vi "newDevice.vi"(8 "error in (no error)":errorcluster, 9 "details":T2, 10 "Device Type":T1=enum."k4b2", 11 "reference in":refnum<class "Devices Controller.lvclass">) -> (0 "error out":errorcluster, 3 "reference out":refnum<class "Devices Controller.lvclass">)   [LabVIEW 2015, in "Devices Controller.lvclass"]
uses:
  Devices Controller.lvclass
  deviceType.ctl
  APP/excelFile_class/fileType.ctl
  APP/k4b2_class/k4b2.lvclass
  APP/rmr_class/rmr.lvclass
  APP/fitmate_class/fitmate.lvclass
  APP/cpet_class/cpet.lvclass
  APP/bodpod_class/bodpod.lvclass
  APP/peapod_class/peapod.lvclass
  APP/excelFile_class/excelFile.lvclass
  File Controller_llb/File Controller.lvclass
  APP/k5_class/k5.lvclass
  APP/bb-pft_class/bb-pft.lvclass
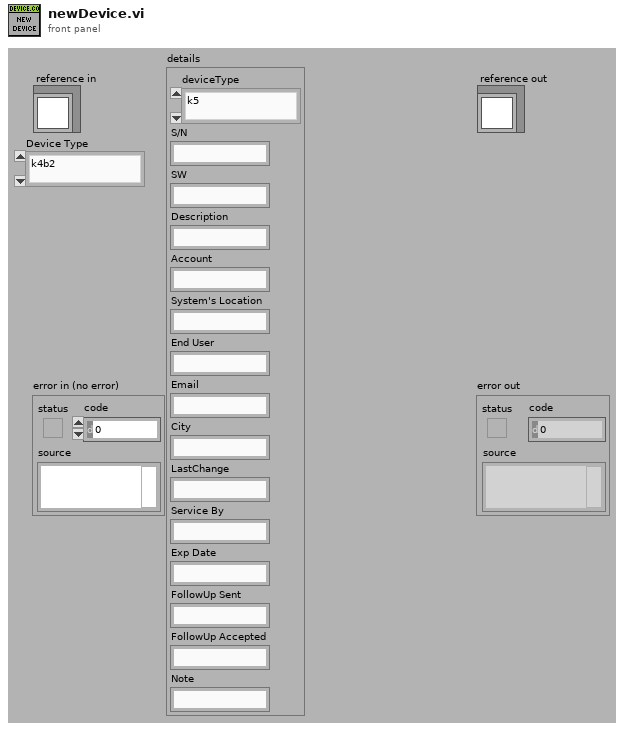
[diagram p1: front panel]
types:
  T1 = typedef "Devices Controller.lvclass/deviceType.ctl" = enum16{"k5", "k4b2", "fitmate", "cpet", "rmr", "bodyBoxPft", "bp", "pp"}
  T2 = cluster{"deviceType":T1, "S/N":string, "SW":string, "Description":string, "Account":string, "System's Location":string, "End User":string, "Email":string, "City":string, "LastChange":string, "Service By":string, "Exp Date":string, "FollowUp Sent":string, "FollowUp Accepted":string, "Note":string}
  T3 = typedef "excelFile.lvclass/fileType.ctl" = enum16{"devices", "items", "partsTracking"}
  T4 = cluster{"deviceType":T1, "S/N":string, "SW":string, "Description":string, "Account":string, "System's Location":string, "End User":string, "Email":string, "City":string, "FollowUp Sent":string, "FollowUp Accepted":string, "Note":string}
  T5 = typedef "Devices Controller.lvclass/ObjectAttributesRef.ctl" = refnum<data-value>
  T6 = typedef "Devices Controller.lvclass/ObjectAttributes.ctl" = cluster{"MyAttribute":dbl, "file_controller_ref":refnum<class "File Controller.lvclass">, "data":string[][][], "devices_refs":cluster{"k4b2_refs":refnum<class "k4b2.lvclass">[], "rmr_refs":refnum<class "rmr.lvclass">[], "bod_pod_refs":refnum<class "bodpod.lvclass">[], "cpet_refs":refnum<class "cpet.lvclass">[], "fitmate_refs":refnum<class "fitmate.lvclass">[], "pea_pod_refs":refnum<class "peapod.lvclass">[], "k5_refs":refnum<class "k5.lvclass">[], "bb-pft_refs":refnum<class "bb-pft.lvclass">[]}}
  T7 = cluster{"k4b2_refs":refnum<class "k4b2.lvclass">[], "rmr_refs":refnum<class "rmr.lvclass">[], "bod_pod_refs":refnum<class "bodpod.lvclass">[], "cpet_refs":refnum<class "cpet.lvclass">[], "fitmate_refs":refnum<class "fitmate.lvclass">[], "pea_pod_refs":refnum<class "peapod.lvclass">[], "k5_refs":refnum<class "k5.lvclass">[], "bb-pft_refs":refnum<class "bb-pft.lvclass">[]}
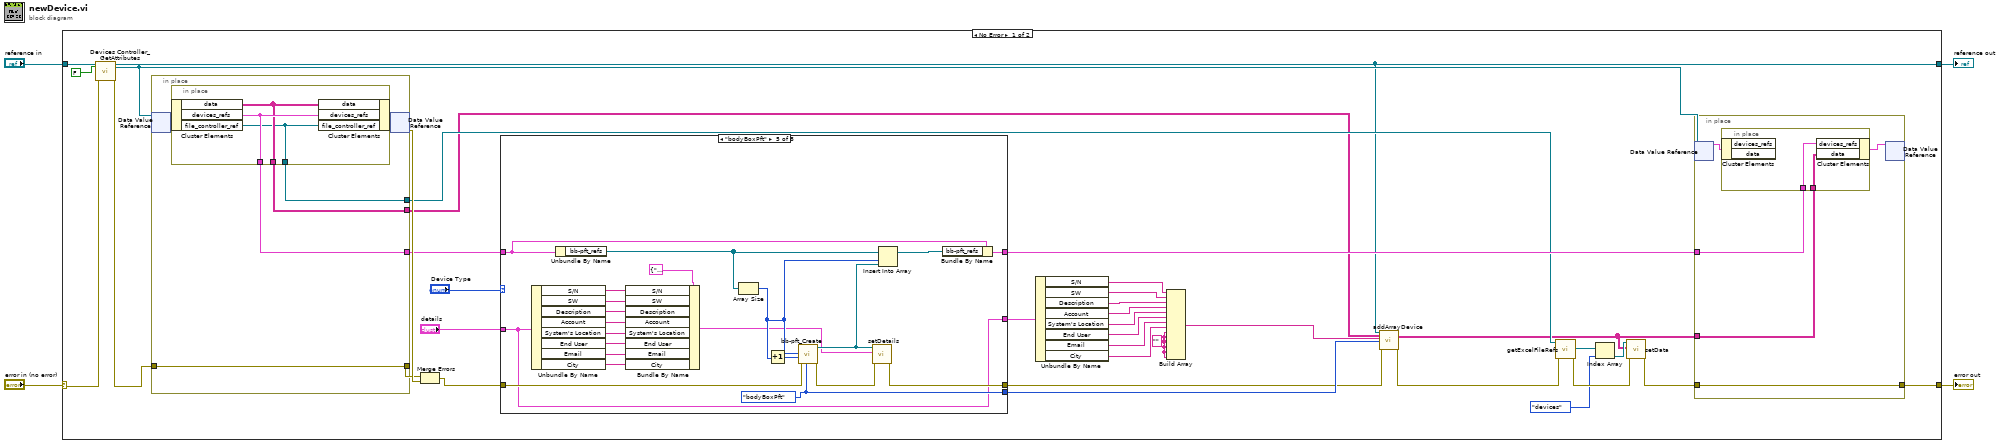
[diagram p0: block diagram]
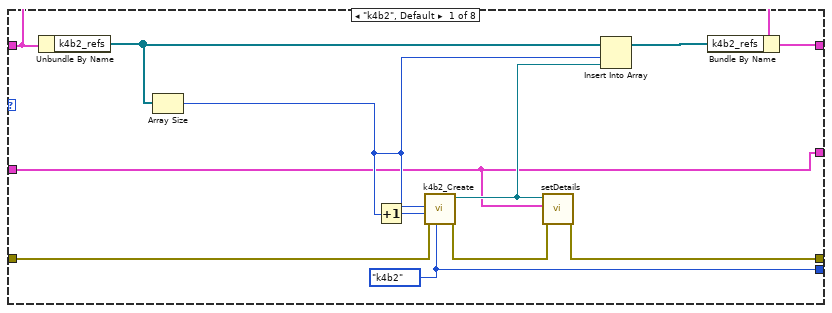
[diagram p2: hidden frame]
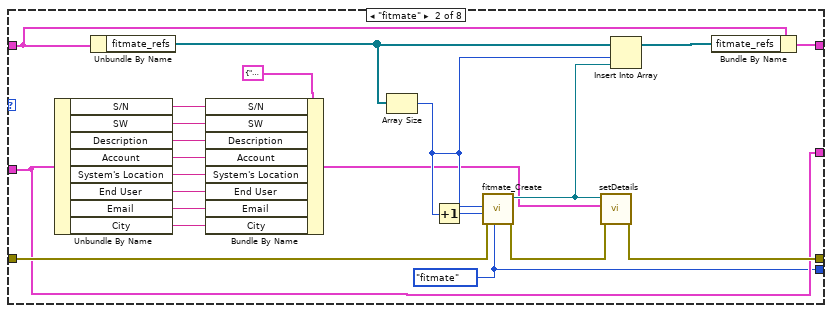
[diagram p3: hidden frame]
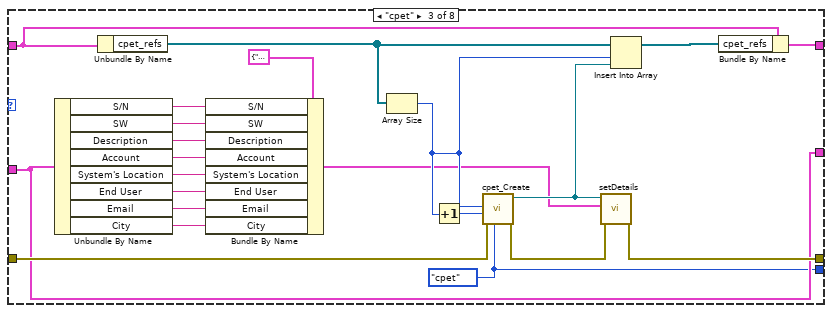
[diagram p4: hidden frame]
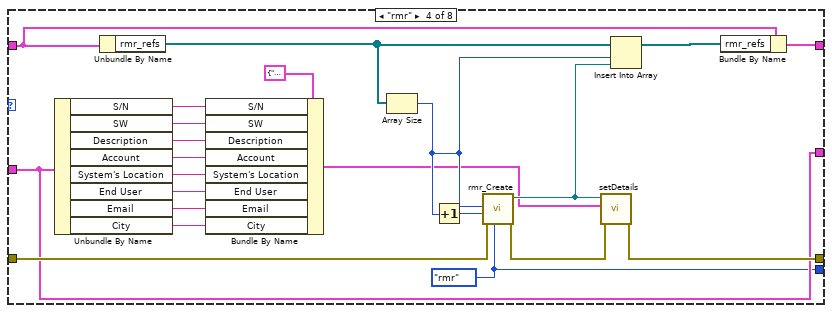
[diagram p5: hidden frame]
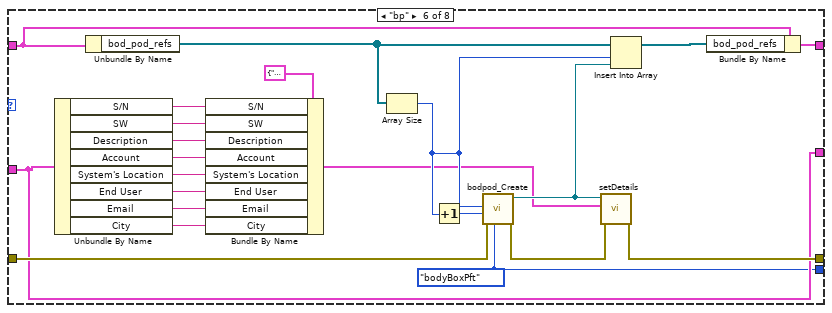
[diagram p6: hidden frame]
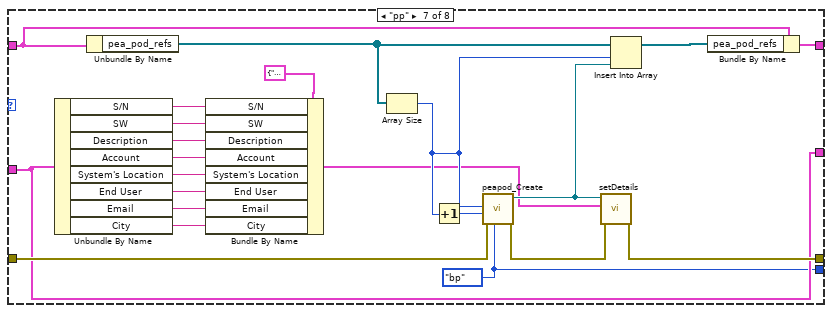
[diagram p7: hidden frame]
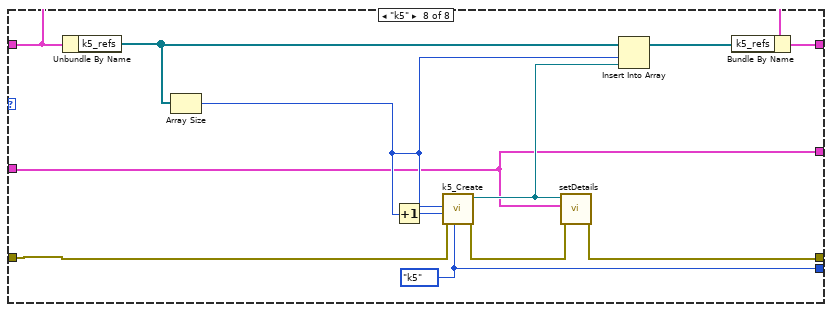
[diagram p8: hidden frame]
diagram:
  n1 = case shown="No Error" "error in (no error)" {
    selector: "error in (no error)" -> [w36 w214]
    tunnel: [w31 w214] -> w3
    tunnel: [w5 w213] -> w1
    tunnel: "reference in" -> [w38 w213]
    frame No Error {
      w10 = "" ("City")
      n2 = call "Devices Controller_GetAttributes.vi"("reference in"=w38, "return data? (T)"=FALSE, "error in (no error)"=w36) -> ("reference out"=w5:refnum<class "Devices Controller.lvclass">, "attributes ref"=w30:T5, "error out"=w32:errorcluster)  [unwired: 13 in, 1 out]
      n3 = in-place {
        in-place-border: w32 -> [w207]
        in-place-border: [w207] -> w39
        in-place-border: [w206] -> w33
        in-place-border: [w205] -> w9
        in-place-border: [w204] -> w14
        n4 = in-place-dvr #1(w30) -> (w208:T6)  [unwired: 1 out]
        n5 = in-place {
          in-place-border: [w212] -> w206
          in-place-border: [w211] -> w205
          in-place-border: [w210] -> w204
          n6 = in-place-cluster #2(w208) -> ("data"=w211:string[][][], "devices_refs"=w212:T7, "file_controller_ref"=w210:refnum<class "File Controller.lvclass">)
          n7 = in-place-cluster #2("data"=w211, "devices_refs"=w212, "file_controller_ref"=w210) -> (w209:T6)
        }
        n8 = in-place-dvr #1(w209) -> (w40:errorcluster)  [unwired: 1 out]
      }
      n9 = Merge Errors(w39, w40) -> (w35:errorcluster)
      n10 = case shown="\"bodyBoxPft\"" "Device Type" {
        tunnel: w35 -> [w59 w75 w97 w119 w132 w163 w185 w197]
        tunnel: [w50 w74 w96 w118 w130 w162 w184 w196] -> w7
        tunnel: "details" -> [w48 w63 w85 w107 w126 w151 w173 w195]
        tunnel: w33 -> [w56 w72 w94 w116 w131 w160 w182 w198]
        tunnel: [w51 w73 w95 w117 w129 w161 w183 w194] -> w29
        tunnel: [w48 w63 w85 w107 w126 w151 w173 w195] -> w17
        tunnel: [w49 w62 w84 w106 w127 w150 w172 w193] -> w11
        frame "k4b2", Default {
          w49 = deviceType."k4b2" ("deviceType")
          n11 = Unbundle By Name(w56) -> ("k4b2_refs"=w55:refnum<class "k4b2.lvclass">[])
          n12 = Array Size(array=w55) -> (size(s)=w52:i32)
          n13 = Increment(x=w52) -> (x+1=w58:i32)
          n14 = call "k4b2_Create.vi"("deviceType"=w49, "error in (no error)"=w59, "dim"=w58, "index"=w52) -> ("error out"=w57:errorcluster, "reference out"=w53:refnum<class "k4b2.lvclass">)  [unwired: 6 in]
          n15 = call "setDetails.vi"("error in (no error)"=w57, "details"=w48, "reference in"=w53) -> ("error out"=w50:errorcluster)  [unwired: 7 in, 1 out]
          n16 = Insert Into Array(array=w55, index=w52, new element=w53) -> (w54:refnum<class "k4b2.lvclass">[])
          n17 = Bundle By Name(cluster=w56, "k4b2_refs"=w54) -> (w51:T7)
        }
        frame "fitmate" {
          w62 = deviceType."fitmate" ("deviceType")
          n18 = Unbundle By Name(w63) -> ("S/N"=w71:string, "SW"=w70:string, "Description"=w69:string, "Account"=w68:string, "System's Location"=w67:string, "End User"=w66:string, "Email"=w65:string, "City"=w64:string)
          n19 = Unbundle By Name(w72) -> ("fitmate_refs"=w79:refnum<class "fitmate.lvclass">[])
          n20 = Bundle By Name(cluster=T4 {"deviceType"=enum."k5", "S/N"="", "SW"="", "Description"="", "Account"="", "System's Location"="", "End User"="", "Email"="", "City"="", "FollowUp Sent"="", "FollowUp Accepted"="", "Note"=""} ("details"), "S/N"=w71, "SW"=w70, "Description"=w69, "Account"=w68, "System's Location"=w67, "End User"=w66, "Email"=w65, "City"=w64) -> (w60:T4)
          n21 = Array Size(array=w79) -> (size(s)=w76:i32)
          n22 = Increment(x=w76) -> (x+1=w81:i32)
          n23 = call "fitmate_Create.vi"("deviceType"=w62, "error in (no error)"=w75, "dim"=w81, "index"=w76) -> ("error out"=w80:errorcluster, "reference out"=w77:refnum<class "fitmate.lvclass">)  [unwired: 6 in]
          n24 = call "setDetails.vi"("error in (no error)"=w80, "details"=w60, "reference in"=w77) -> ("error out"=w74:errorcluster)  [unwired: 7 in, 1 out]
          n25 = Insert Into Array(array=w79, index=w76, new element=w77) -> (w78:refnum<class "fitmate.lvclass">[])
          n26 = Bundle By Name(cluster=w72, "fitmate_refs"=w78) -> (w73:T7)
        }
        frame "cpet" {
          w84 = deviceType."cpet" ("deviceType")
          n27 = Unbundle By Name(w85) -> ("S/N"=w93:string, "SW"=w92:string, "Description"=w91:string, "Account"=w90:string, "System's Location"=w89:string, "End User"=w88:string, "Email"=w87:string, "City"=w86:string)
          n28 = Unbundle By Name(w94) -> ("cpet_refs"=w101:refnum<class "cpet.lvclass">[])
          n29 = Bundle By Name(cluster=T4 {"deviceType"=enum."k5", "S/N"="", "SW"="", "Description"="", "Account"="", "System's Location"="", "End User"="", "Email"="", "City"="", "FollowUp Sent"="", "FollowUp Accepted"="", "Note"=""} ("details"), "S/N"=w93, "SW"=w92, "Description"=w91, "Account"=w90, "System's Location"=w89, "End User"=w88, "Email"=w87, "City"=w86) -> (w82:T4)
          n30 = Array Size(array=w101) -> (size(s)=w98:i32)
          n31 = Increment(x=w98) -> (x+1=w103:i32)
          n32 = call "cpet_Create.vi"("deviceType"=w84, "error in (no error)"=w97, "dim"=w103, "index"=w98) -> ("error out"=w102:errorcluster, "reference out"=w99:refnum<class "cpet.lvclass">)  [unwired: 6 in]
          n33 = call "setDetails.vi"("error in (no error)"=w102, "details"=w82, "reference in"=w99) -> ("error out"=w96:errorcluster)  [unwired: 7 in, 1 out]
          n34 = Insert Into Array(array=w101, index=w98, new element=w99) -> (w100:refnum<class "cpet.lvclass">[])
          n35 = Bundle By Name(cluster=w94, "cpet_refs"=w100) -> (w95:T7)
        }
        frame "rmr" {
          w106 = deviceType."rmr" ("deviceType")
          n36 = Unbundle By Name(w107) -> ("S/N"=w115:string, "SW"=w114:string, "Description"=w113:string, "Account"=w112:string, "System's Location"=w111:string, "End User"=w110:string, "Email"=w109:string, "City"=w108:string)
          n37 = Unbundle By Name(w116) -> ("rmr_refs"=w123:refnum<class "rmr.lvclass">[])
          n38 = Bundle By Name(cluster=T4 {"deviceType"=enum."k5", "S/N"="", "SW"="", "Description"="", "Account"="", "System's Location"="", "End User"="", "Email"="", "City"="", "FollowUp Sent"="", "FollowUp Accepted"="", "Note"=""} ("details"), "S/N"=w115, "SW"=w114, "Description"=w113, "Account"=w112, "System's Location"=w111, "End User"=w110, "Email"=w109, "City"=w108) -> (w104:T4)
          n39 = Array Size(array=w123) -> (size(s)=w120:i32)
          n40 = Increment(x=w120) -> (x+1=w125:i32)
          n41 = call "rmr_Create.vi"("deviceType"=w106, "error in (no error)"=w119, "dim"=w125, "index"=w120) -> ("error out"=w124:errorcluster, "reference out"=w121:refnum<class "rmr.lvclass">)  [unwired: 6 in]
          n42 = call "setDetails.vi"("error in (no error)"=w124, "details"=w104, "reference in"=w121) -> ("error out"=w118:errorcluster)  [unwired: 7 in, 1 out]
          n43 = Insert Into Array(array=w123, index=w120, new element=w121) -> (w122:refnum<class "rmr.lvclass">[])
          n44 = Bundle By Name(cluster=w116, "rmr_refs"=w122) -> (w117:T7)
        }
        frame "bodyBoxPft" {
          w127 = deviceType."bodyBoxPft" ("deviceType")
          n45 = Unbundle By Name(w126) -> ("S/N"=w141:string, "SW"=w140:string, "Description"=w139:string, "Account"=w138:string, "System's Location"=w137:string, "End User"=w136:string, "Email"=w135:string, "City"=w134:string)
          n46 = Unbundle By Name(w131) -> ("bb-pft_refs"=w145:refnum<class "bb-pft.lvclass">[])
          n47 = Bundle By Name(cluster=T4 {"deviceType"=enum."k5", "S/N"="", "SW"="", "Description"="", "Account"="", "System's Location"="", "End User"="", "Email"="", "City"="", "FollowUp Sent"="", "FollowUp Accepted"="", "Note"=""} ("details"), "S/N"=w141, "SW"=w140, "Description"=w139, "Account"=w138, "System's Location"=w137, "End User"=w136, "Email"=w135, "City"=w134) -> (w128:T4)
          n48 = Array Size(array=w145) -> (size(s)=w142:i32)
          n49 = Increment(x=w142) -> (x+1=w147:i32)
          n50 = call "bb-pft_Create.vi"("deviceType"=w127, "error in (no error)"=w132, "dim"=w147, "index"=w142) -> ("error out"=w146:errorcluster, "reference out"=w143:refnum<class "bb-pft.lvclass">)  [unwired: 6 in]
          n51 = call "setDetails.vi"("error in (no error)"=w146, "details"=w128, "reference in"=w143) -> ("error out"=w130:errorcluster)  [unwired: 7 in, 1 out]
          n52 = Insert Into Array(array=w145, index=w142, new element=w143) -> (w144:refnum<class "bb-pft.lvclass">[])
          n53 = Bundle By Name(cluster=w131, "bb-pft_refs"=w144) -> (w129:T7)
        }
        frame "bp" {
          w150 = deviceType."bodyBoxPft" ("deviceType")
          n54 = Unbundle By Name(w151) -> ("S/N"=w159:string, "SW"=w158:string, "Description"=w157:string, "Account"=w156:string, "System's Location"=w155:string, "End User"=w154:string, "Email"=w153:string, "City"=w152:string)
          n55 = Unbundle By Name(w160) -> ("bod_pod_refs"=w167:refnum<class "bodpod.lvclass">[])
          n56 = Bundle By Name(cluster=T4 {"deviceType"=enum."k5", "S/N"="", "SW"="", "Description"="", "Account"="", "System's Location"="", "End User"="", "Email"="", "City"="", "FollowUp Sent"="", "FollowUp Accepted"="", "Note"=""} ("details"), "S/N"=w159, "SW"=w158, "Description"=w157, "Account"=w156, "System's Location"=w155, "End User"=w154, "Email"=w153, "City"=w152) -> (w148:T4)
          n57 = Array Size(array=w167) -> (size(s)=w164:i32)
          n58 = Increment(x=w164) -> (x+1=w169:i32)
          n59 = call "bodpod_Create.vi"("deviceType"=w150, "error in (no error)"=w163, "dim"=w169, "index"=w164) -> ("error out"=w168:errorcluster, "reference out"=w165:refnum<class "bodpod.lvclass">)  [unwired: 6 in]
          n60 = call "setDetails.vi"("error in (no error)"=w168, "details"=w148, "reference in"=w165) -> ("error out"=w162:errorcluster)  [unwired: 7 in, 1 out]
          n61 = Insert Into Array(array=w167, index=w164, new element=w165) -> (w166:refnum<class "bodpod.lvclass">[])
          n62 = Bundle By Name(cluster=w160, "bod_pod_refs"=w166) -> (w161:T7)
        }
        frame "pp" {
          w172 = deviceType."bp" ("deviceType")
          n63 = Unbundle By Name(w173) -> ("S/N"=w181:string, "SW"=w180:string, "Description"=w179:string, "Account"=w178:string, "System's Location"=w177:string, "End User"=w176:string, "Email"=w175:string, "City"=w174:string)
          n64 = Unbundle By Name(w182) -> ("pea_pod_refs"=w189:refnum<class "peapod.lvclass">[])
          n65 = Bundle By Name(cluster=T4 {"deviceType"=enum."k5", "S/N"="", "SW"="", "Description"="", "Account"="", "System's Location"="", "End User"="", "Email"="", "City"="", "FollowUp Sent"="", "FollowUp Accepted"="", "Note"=""} ("details"), "S/N"=w181, "SW"=w180, "Description"=w179, "Account"=w178, "System's Location"=w177, "End User"=w176, "Email"=w175, "City"=w174) -> (w170:T4)
          n66 = Array Size(array=w189) -> (size(s)=w186:i32)
          n67 = Increment(x=w186) -> (x+1=w191:i32)
          n68 = call "peapod_Create.vi"("deviceType"=w172, "error in (no error)"=w185, "dim"=w191, "index"=w186) -> ("error out"=w190:errorcluster, "reference out"=w187:refnum<class "peapod.lvclass">)  [unwired: 6 in]
          n69 = call "setDetails.vi"("error in (no error)"=w190, "details"=w170, "reference in"=w187) -> ("error out"=w184:errorcluster)  [unwired: 7 in, 1 out]
          n70 = Insert Into Array(array=w189, index=w186, new element=w187) -> (w188:refnum<class "peapod.lvclass">[])
          n71 = Bundle By Name(cluster=w182, "pea_pod_refs"=w188) -> (w183:T7)
        }
        frame "k5" {
          w193 = deviceType."k5" ("deviceType")
          n72 = Unbundle By Name(w198) -> ("k5_refs"=w201:refnum<class "k5.lvclass">[])
          n73 = Array Size(array=w201) -> (size(s)=w199:i32)
          n74 = Increment(x=w199) -> (x+1=w203:i32)
          n75 = call "k5_Create.vi"("deviceType"=w193, "error in (no error)"=w197, "dim"=w203, "index"=w199) -> ("error out"=w202:errorcluster, "reference out"=w200:refnum<class "k5.lvclass">)  [unwired: 6 in]
          n76 = call "setDetails.vi"("error in (no error)"=w202, "details"=w195, "reference in"=w200) -> ("error out"=w196:errorcluster)  [unwired: 7 in, 1 out]
          n77 = Insert Into Array(array=w201, index=w199, new element=w200) -> (w192:refnum<class "k5.lvclass">[])
          n78 = Bundle By Name(cluster=w198, "k5_refs"=w192) -> (w194:T7)
        }
      }
      n79 = Unbundle By Name(w17) -> ("S/N"=w28:string, "SW"=w27:string, "Description"=w26:string, "Account"=w25:string, "System's Location"=w24:string, "End User"=w23:string, "Email"=w22:string, "City"=w21:string)
      n80 = Build Array(w28, w27, w26, w25, w24, w23, w22, w21, w10, w10, w10, w10, w10, w10) -> (w12:string[])
      n81 = call "addArrayDevice.vi"("reference in"=w5, "data in"=w9, "Array"=w12, "deviceType"=w11, "error in (no error)"=w7) -> ("data out"=w8:string[][][], "error out"=w6:errorcluster)  [unwired: 12 in, 1 out]
      n82 = call "getExcelFileRefs.vi"("error in (no error)"=w6, "reference in"=w14) -> ("error out"=w20:errorcluster, "excelFile_refs"=w19:refnum<class "excelFile.lvclass">[])  [unwired: 7 in, 1 out]
      n83 = Index Array(array=w19, index=fileType."devices" ("fileType")) -> (element=w18:refnum<class "excelFile.lvclass">)
      n84 = call "setData.vi"("error in (no error)"=w20, "data"=w8, "reference in"=w18) -> ("error out"=w15:errorcluster)  [unwired: 7 in, 1 out]
      n85 = in-place {
        in-place-border: w15 -> [w43]
        in-place-border: [w43] -> w31
        in-place-border: w29 -> [w42]
        in-place-border: w8 -> [w41]
        n86 = in-place-dvr #3(w30) -> (w44:T6)  [unwired: 1 out]
        n87 = in-place {
          in-place-border: w42 -> [w47]
          in-place-border: w41 -> [w46]
          n88 = in-place-cluster #4(w44) -> ()  [unwired: 2 out]
          n89 = in-place-cluster #4("devices_refs"=w47, "data"=w46) -> (w45:T6)
        }
        n90 = in-place-dvr #3(w45) -> ()  [unwired: 2 out]
      }
    }
    frame Error {
    }
  }
  "error out" <- w3
  "reference out" <- w1
